vi "Add content to Engine library.vi"(6 "Project Name":string, 8 "error in":errorcluster, 9 "Project Root":path, 10 "CD Wizard - Internal Data":T1, 11 "CD Template":refnum<class "NIVS_PPL_Inline HW Interface (Inline-Async).lvclass">) -> (0 "error out":errorcluster)   [LabVIEW 2020, in "NIVS_PPL_Inline HW Interface (Inline-Async).lvclass"]
doc: "Add all virtual folders and VIs to the Engine library."
uses:
  NIVS_PPL_Inline HW Interface (Inline-Async).lvclass
  NIVS_Consolidated_CDW_MetaDataObj/Internal data.ctl
  C:/dev/Karthick/FPGA Addons Packages/niveristand-custom-device-wizard/ProjectTemplate/Source/NI VeriStand/Custom Device/Template Classes/NIVS_CD Template/NIVS_CD Template.lvclass
  NIVS_Consolidated_CDW_MetaDataObj/CD Engine lvlib.ctl
  NIVS_Consolidated_CDW_MetaDataObj/Add Item - Type.ctl
  NIVS_CD Template/NIVS_CD Template.lvclass/NIVS_CD Template.ctl
  NIVS_Consolidated_CDW_MetaDataObj/CD Engine lvlib.vi
  NIVS_Consolidated_CDW_MetaDataObj/NIVS_Consolidated_CDW_MetaDataObj.lvclass
  NIVS_CD Template/NIVS_CD Template.lvclass
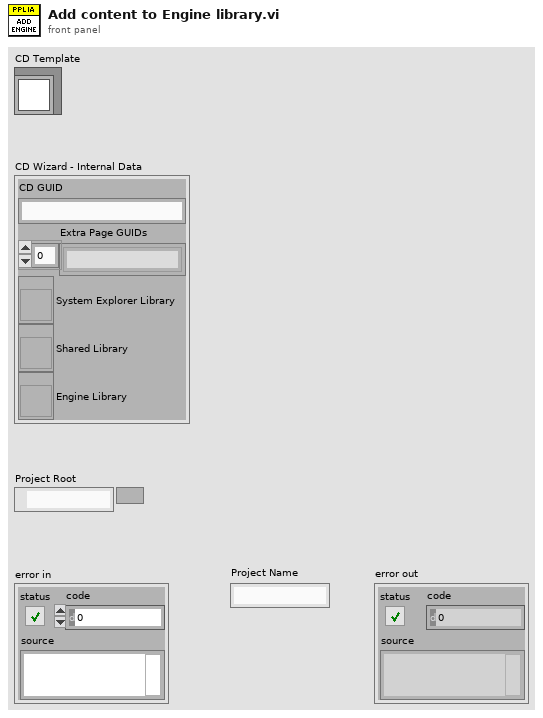
[diagram p1: front panel]
types:
  T1 = typedef "NIVS_Consolidated_CDW_MetaDataObj.lvclass/Internal data.ctl" = cluster{"CD GUID":string, "Extra Page GUIDs":string[], "System Explorer Library":refnum<vi>, "Shared Library":refnum<vi>, "Engine Library":refnum<vi>}
  T2 = typedef "NIVS_Consolidated_CDW_MetaDataObj.lvclass/CD Engine lvlib.ctl" = enum16{"LibraryFileName", "LibraryFolderName", "Engine.FolderName", "Engine.Init.FolderName", "Engine.Run.FolderName", "Engine.Shutdown.FolderName", "Types.FolderName", "Engine.RT Driver VI.TemplatePath", "Engine.RT Driver VI.FileName", "Engine.PPL.RT Driver VI_InlineAsync.FileName", "Engine.RTStateVariables.Name", "Engine.PPL.RTStateVariables.Name", "Engine.RTStateVariables.Name.NoExtension", "Engine.Async.NameExtension", "Engine.Async.TemplateName", "Engine.PPL.Async.TemplateName", "Engine.PPL.Async.InitVSGlobals.Name", "Engine.PPL.RT Driver VI_Inline.FileName", "Engine.LaunchCommandLoop.Name", "Engine.CommandLoop.Name"}
  T3 = typedef "NIVS_Consolidated_CDW_MetaDataObj.lvclass/Add Item - Type.ctl" = string
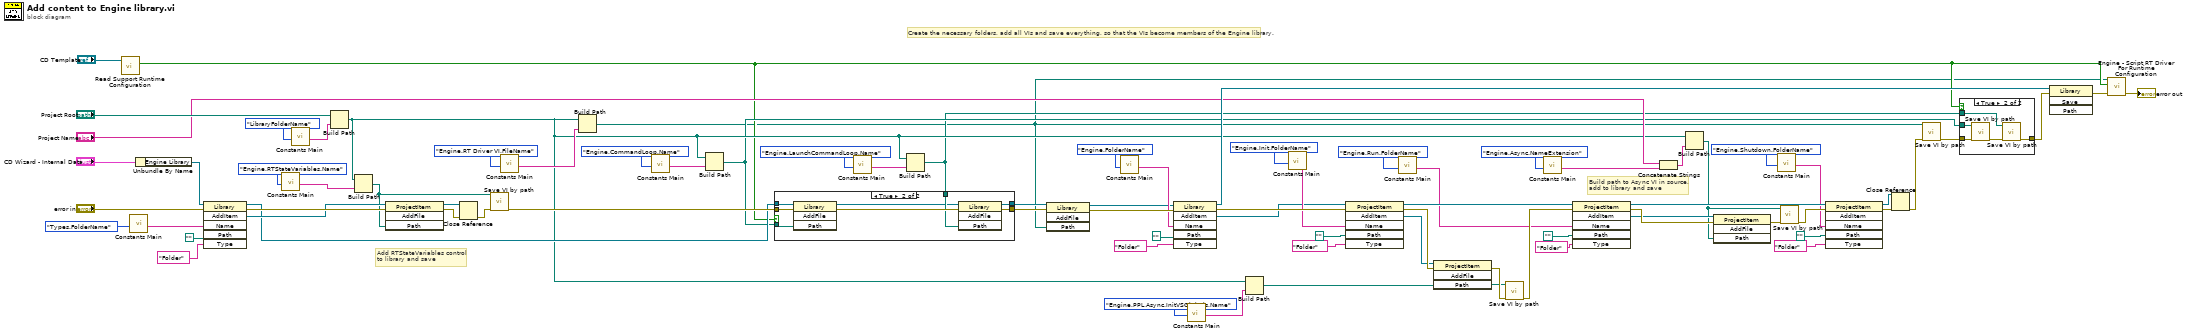
[diagram p0: block diagram]
diagram:
  # "Create the necessary folders, add all VIs and save everything, so that the VIs become members of the Engine library."
  # "Add RTStateVariables control\nto library and save"
  # "Build path to Async VI in source,\nadd to library and save"
  n1 = call "Read Support Runtime Configuration.vi"("NIVS_CD Template in"="CD Template") -> ("Support Runtime Configuration"=w2:bool)  [unwired: 8 in, 2 out]
  n2 = call-poly "Constants Main.vi"("Action"=CD_Engine_lvlib."Types.FolderName") -> ("Output"=w59:string)  [unwired: 10 in]
  n3 = Unbundle By Name("CD Wizard - Internal Data") -> ("Engine Library"=w49:refnum<vi>)
  n4 = invoke class="Library" method="AddItem"(reference=w49, error in="error in", "Name"=w59, "Path"=path "", "Type"=T3 "Folder" ("Add Item - Type")) -> (reference out=w21:refnum<vi>, error out=w75:errorcluster, "AddItem"=w30:refnum<vi>)  [unwired: 1 in, 3 out]
  n5 = call-poly "Constants Main.vi"("Action"=CD_Engine_lvlib."Engine.RTStateVariables.Name") -> ("Output"=w22:string)  [unwired: 10 in]
  n6 = call-poly "Constants Main.vi"("Action"=CD_Engine_lvlib."LibraryFolderName") -> ("Output"=w51:string)  [unwired: 10 in]
  n7 = Build Path(base path="Project Root", name or relative path=w51) -> (appended path=w8:path)
  n8 = Build Path(base path=w8, name or relative path=w22) -> (appended path=w29:path)
  n9 = invoke class="ProjectItem" method="AddFile"(reference=w30, error in=w75, "Path"=w29) -> (reference out=w20:refnum<vi>, error out=w78:errorcluster)  [unwired: 1 in, 2 out]
  n10 = Close Reference(reference=w20, error in (no error)=w78) -> (error out=w73:errorcluster)
  n11 = call "Save VI by path.vi"("error in (no error)"=w73, "VI path"=w29) -> ("error out"=w74:errorcluster)  [unwired: 9 in]
  n12 = call-poly "Constants Main.vi"("Action"=CD_Engine_lvlib."Engine.RT Driver VI.FileName") -> ("Output"=w53:string)  [unwired: 10 in]
  n13 = Build Path(base path=w8, name or relative path=w53) -> (appended path=w1:path)
  n14 = call-poly "Constants Main.vi"("Action"=CD_Engine_lvlib."Engine.CommandLoop.Name") -> ("Output"=w10:string)  [unwired: 10 in]
  n15 = Build Path(base path=w8, name or relative path=w10) -> (appended path=w6:path)
  n16 = call-poly "Constants Main.vi"("Action"=CD_Engine_lvlib."Engine.LaunchCommandLoop.Name") -> ("Output"=w9:string)  [unwired: 10 in]
  n17 = Build Path(base path=w8, name or relative path=w9) -> (appended path=w5:path)
  n18 = case shown="True" w2 {
    tunnel: w21 -> [w81 w87]
    tunnel: w6 -> [_ w86]
    tunnel: w5 -> [_ w85]
    tunnel: [w81 w83] -> w4
    tunnel: [w82 w89] -> w64
    tunnel: w74 -> [w82 w88]
    frame False {
    }
    frame True {
      n19 = invoke class="Library" method="AddFile"(reference=w87, error in=w88, "Path"=w86) -> (reference out=w84:refnum<vi>, error out=w90:errorcluster)  [unwired: 1 in, 2 out]
      n20 = invoke class="Library" method="AddFile"(reference=w84, error in=w90, "Path"=w85) -> (reference out=w83:refnum<vi>, error out=w89:errorcluster)  [unwired: 1 in, 2 out]
    }
  }
  n21 = invoke class="Library" method="AddFile"(reference=w4, error in=w64, "Path"=w1) -> (reference out=w3:refnum<vi>, error out=w63:errorcluster)  [unwired: 1 in, 2 out]
  n22 = call-poly "Constants Main.vi"("Action"=CD_Engine_lvlib."Engine.FolderName") -> ("Output"=w46:string)  [unwired: 10 in]
  n23 = invoke class="Library" method="AddItem"(reference=w3, error in=w63, "Name"=w46, "Path"=path "", "Type"=T3 "Folder" ("Add Item - Type")) -> (reference out=w33:refnum<vi>, error out=w72:errorcluster, "AddItem"=w44:refnum<vi>)  [unwired: 1 in, 3 out]
  n24 = call-poly "Constants Main.vi"("Action"=CD_Engine_lvlib."Engine.PPL.Async.InitVSGlobals.Name") -> ("Output"=w15:string)  [unwired: 10 in]
  n25 = Build Path(base path=w8, name or relative path=w15) -> (appended path=w13:path)
  n26 = call-poly "Constants Main.vi"("Action"=CD_Engine_lvlib."Engine.Init.FolderName") -> ("Output"=w55:string)  [unwired: 10 in]
  n27 = invoke class="ProjectItem" method="AddItem"(reference=w44, error in=w72, "Name"=w55, "Path"=path "", "Type"=T3 "Folder" ("Add Item - Type")) -> (reference out=w42:refnum<vi>, error out=w69:errorcluster, "AddItem"=w14:refnum<vi>)  [unwired: 1 in, 3 out]
  n28 = call-poly "Constants Main.vi"("Action"=CD_Engine_lvlib."Engine.Run.FolderName") -> ("Output"=w40:string)  [unwired: 10 in]
  n29 = invoke class="ProjectItem" method="AddFile"(reference=w14, error in=w69, "Path"=w13) -> (error out=w68:errorcluster)  [unwired: 1 in, 3 out]
  n30 = call "Save VI by path.vi"("error in (no error)"=w68, "VI path"=w13) -> ("error out"=w67:errorcluster)  [unwired: 9 in]
  n31 = call-poly "Constants Main.vi"("Action"=CD_Engine_lvlib."Engine.Async.NameExtension") -> ("Output"=w24:string)  [unwired: 10 in]
  n32 = invoke class="ProjectItem" method="AddItem"(reference=w42, error in=w67, "Name"=w40, "Path"=path "", "Type"=T3 "Folder" ("Add Item - Type")) -> (reference out=w34:refnum<vi>, error out=w77:errorcluster, "AddItem"=w28:refnum<vi>)  [unwired: 1 in, 3 out]
  n33 = Concatenate Strings("Project Name", w24) -> (w27:string)
  n34 = Build Path(base path=w8, name or relative path=w27) -> (appended path=w26:path)
  n35 = invoke class="ProjectItem" method="AddFile"(reference=w28, error in=w77, "Path"=w26) -> (error out=w76:errorcluster)  [unwired: 1 in, 3 out]
  n36 = call-poly "Constants Main.vi"("Action"=CD_Engine_lvlib."Engine.Shutdown.FolderName") -> ("Output"=w32:string)  [unwired: 10 in]
  n37 = call "Save VI by path.vi"("error in (no error)"=w76, "VI path"=w26) -> ("error out"=w71:errorcluster)  [unwired: 9 in]
  n38 = invoke class="ProjectItem" method="AddItem"(reference=w34, error in=w71, "Name"=w32, "Path"=path "", "Type"=T3 "Folder" ("Add Item - Type")) -> (reference out=w31:refnum<vi>, error out=w80:errorcluster)  [unwired: 1 in, 4 out]
  n39 = Close Reference(reference=w31, error in (no error)=w80) -> (error out=w79:errorcluster)
  n40 = call "Save VI by path.vi"("error in (no error)"=w79, "VI path"=w1) -> ("error out"=w66:errorcluster)  [unwired: 9 in]
  n41 = case shown="True" w2 {
    tunnel: w66 -> [w91 w96]
    tunnel: w6 -> [_ w93]
    tunnel: w5 -> [_ w92]
    tunnel: [w91 w94] -> w65
    frame False {
    }
    frame True {
      n42 = call "Save VI by path.vi"("error in (no error)"=w96, "VI path"=w93) -> ("error out"=w95:errorcluster)  [unwired: 9 in]
      n43 = call "Save VI by path.vi"("error in (no error)"=w95, "VI path"=w92) -> ("error out"=w94:errorcluster)  [unwired: 9 in]
    }
  }
  n44 = invoke class="Library" method="Save"(reference=w33, error in=w65) -> (error out=w62:errorcluster)  [unwired: 2 in, 3 out]
  n45 = call "Engine - Script RT Driver For Runtime Configuration.vi"("error in"=w62, "Support Runtime Configuration"=w2, "RT Driver VI Path"=w1) -> ("error out"=→"error out":errorcluster)  [unwired: 8 in]
